vi "MaskArrayValue.vi"(1 "Array In":u32[][](array[numeric])) -> (0 "Array out":u32[][](array[numeric]))   [LabVIEW 2020, in "test.lvlib" / "01_Image.lvclass"]
uses:
  01_Image.lvclass
  01_Image.lvclass/01_Image.ctl
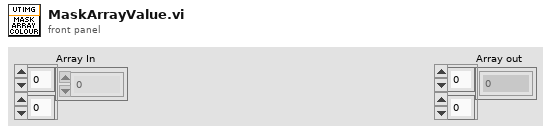
[diagram p1: front panel]
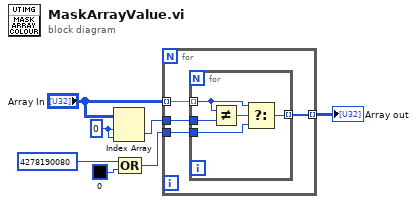
[diagram p0: block diagram]
diagram:
  w2 = 0 ("index (row)")
  n1 = Index Array(array="Array In", index (row)=w2, index (col)=w2) -> (element=w1:u32)
  n2 = Compound Arithmetic op=OR(u32 4278190080, u32 0 ("Replace With")) -> (w6:u32)
  n3 = for {
    tunnel: "Array In" -> [w11] mode=indexing
    tunnel: w1 -> [w10]
    tunnel: [w9] -> w5 mode=indexing
    tunnel: w6 -> [w8]
    n4 = for {
      tunnel: w11 -> [w12] mode=indexing
      tunnel: w10 -> [w15]
      tunnel: [w14] -> w9 mode=indexing
      tunnel: w8 -> [w13]
      n5 = Not Equal?(x=w12, y=w15) -> (x != y?=w16:bool)
      n6 = Select(t=w12, s=w16, f=w13) -> (s? t:f=w14:u32)
    }
  }
  "Array out" <- w5
